vi "Matches.vi"(8 "error in (no error)":errorcluster, 10 "Actual":variant, 11 "Logical And in":refnum<class "Logical And.lvclass">) -> (0 "error out":errorcluster, 2 "Result":bool, 3 "Logical And out":refnum<class "Logical And.lvclass">)   [LabVIEW 2017, in "Transparent Assertions.lvlib" / "Constraints.lvlib" / "Logical And.lvclass"]
doc: "Evaluates the constraint for <B>Actual</B>. Returns true if the constraint is met."
uses:
  Logical And.lvclass
  C:/Users/pasca/Projects/Home/TransparentAssertions/src/Transparent Assertions/Constraints/Binary Operator/Binary Operator.lvclass
  Binary Operator/Binary Operator.lvclass/Binary Operator.ctl
  Binary Operator/Read Constraints.vi
  Constraint/Constraint.lvclass
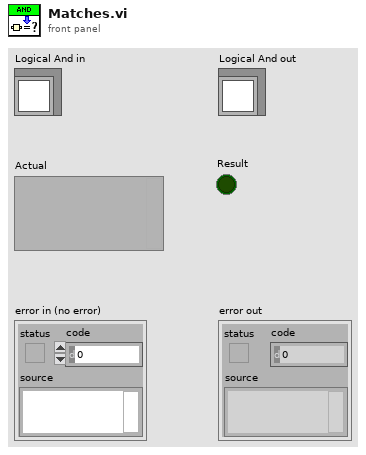
[diagram p1: front panel]
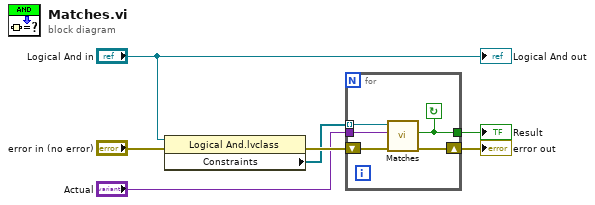
[diagram p0: block diagram]
diagram:
  n1 = property class="Logical And.lvclass"(reference="Logical And in", error in="error in (no error)") -> (error out=w7:errorcluster, "Constraints"=w6:refnum<class "Constraint.lvclass">[])  [unwired: 1 out]
  n2 = for {
    tunnel: w6 -> [w10] mode=indexing
    shift-right: [w11] -> w4
    shift-left: w7 -> [w12]
    tunnel: [w9] -> w1
    tunnel: "Actual" -> [w8]
    stop <- w9 continue-if-true
    n3 = call-dynamic "Matches.vi"("error in (no error)"=w12, "Actual"=w8, "Constraint in"=w10) -> ("error out"=w11:errorcluster, "Result"=w9:bool)  [unwired: 6 in, 1 out]
  }
  "error out" <- w4
  "Result" <- w1
  "Logical And out" <- "Logical And in"
